vi "Drag Location.vi"(8 "error in (no error)":errorcluster, 9 "Coords":T4, 10 "BetterDropOp":refnum<class "BetterDropOp.lvclass">, 11 "Better Tree Handle In":refnum<class "BetterTreeHandle.lvclass">) -> (0 "error out":errorcluster, 2 "DragOver Output":T1={"Displayed Row"=0, "Position"=enum."On Row", "Row's TreeItem index"=0, "indent"=0, "Accepted?"=FALSE, "Insertion index"=0, "Top left visible TreeItem index"=0, "Bar type"=enum."tilda up"}, 3 "Better Tree Handle Out":refnum<class "BetterTreeHandle.lvclass">)   [LabVIEW 2020, in "BetterDragAndDrop.lvlib" / "BetterTreeHandle.lvclass"]
uses:
  BetterTreeHandle.lvclass
  <vilib>/Utility/miscctls.llb/LVPoint32TypeDef.ctl
  SubVIs/DragOver Output.ctl
  SubVIs/DragOverPosition.ctl
  BetterTreeBar/SubVIs/Horizontal Bar Enumeration.ctl
  C:/DSCE code/Open-source/betterdraganddrop_GIT/Source/Classes/BetterHandle/BetterHandle.lvclass
  BetterDropOp/BetterDropOp.lvclass
  BetterHandle/BetterHandle.lvclass/BetterHandle.ctl
  BetterTreeHandle.lvclass/BetterTreeHandle.ctl
  BetterTreeItem/BetterItem.lvclass
  BetterTreeBar/BetterHorizontalBar.lvclass
  BetterHandle/BetterHandle.lvclass
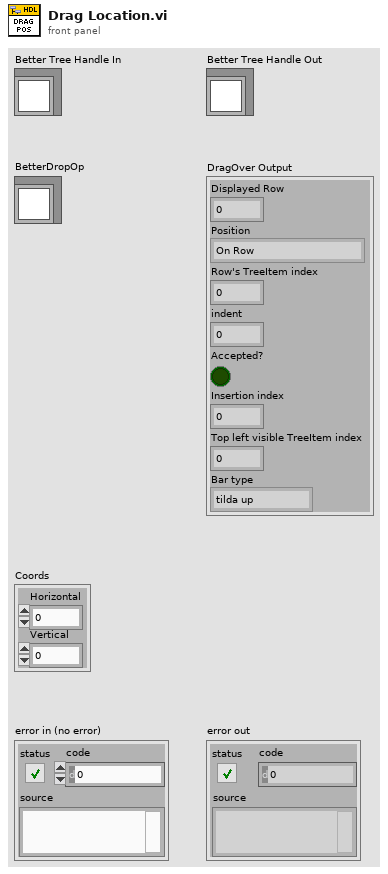
[diagram p1: front panel]
types:
  T1 = typedef "BetterDragAndDrop.lvlib/BetterHandle.lvclass/DragOver Output.ctl" = cluster{"Displayed Row":i32, "Position":T2, "Row's TreeItem index":i32, "indent":i32, "Accepted?":bool, "Insertion index":i32, "Top left visible TreeItem index":i32, "Bar type":T3}
  T2 = typedef "BetterDragAndDrop.lvlib/BetterHandle.lvclass/DragOverPosition.ctl" = enum16{"On Row", "Inbetween"}
  T3 = typedef "BetterDragAndDrop.lvlib/BetterHorizontalBar.lvclass/Horizontal Bar Enumeration.ctl" = enum16{"None", "only bar", "tilda up"}
  T4 = typedef "LVPoint32TypeDef.ctl" = cluster{"Horizontal":i32, "Vertical":i32}
  T5 = typedef "BetterDragAndDrop.lvlib/BetterHandle.lvclass/Pixel Constants.ctl" = cluster{"Row Header height":i32, "Row height":i32, "Column Header Offset":i32}
  T6 = typedef "BetterDragAndDrop.lvlib/BetterTreeHandle.lvclass/TreeItem.ctl" = cluster{"Left Cell String":string, "Child Text":string[], "Child Tag":string, "Item Indent":i32, "Child Only?":bool, "Glyph Index":i32, "Font Color":u32}
  T7 = typedef "LVPositionTypeDef.ctl" = cluster{"Left":i32, "Top":i32}
  T8 = typedef "LVNodeAndColumnTypeDef.ctl" = cluster{"Node":string, "Column":i32}
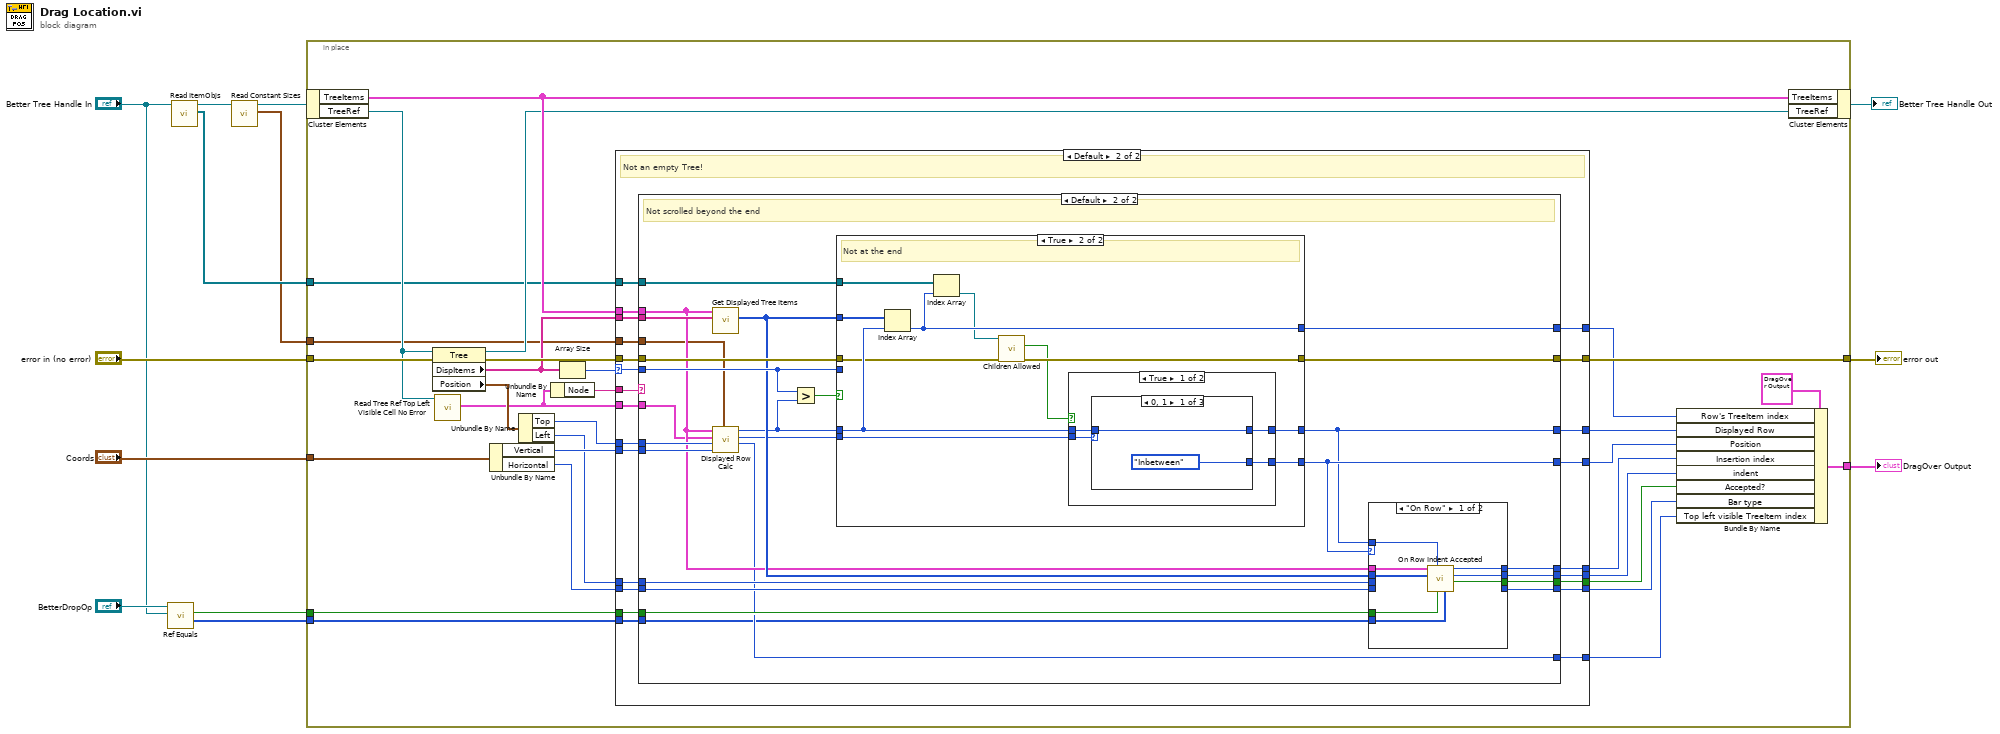
[diagram p0: block diagram]
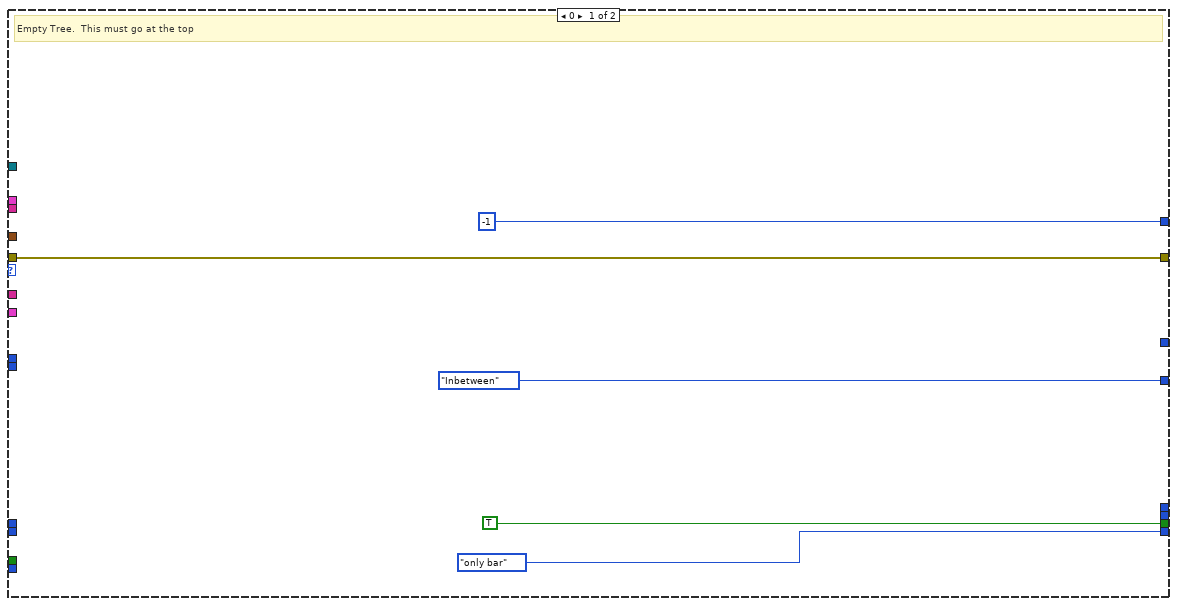
[diagram p2: hidden frame]
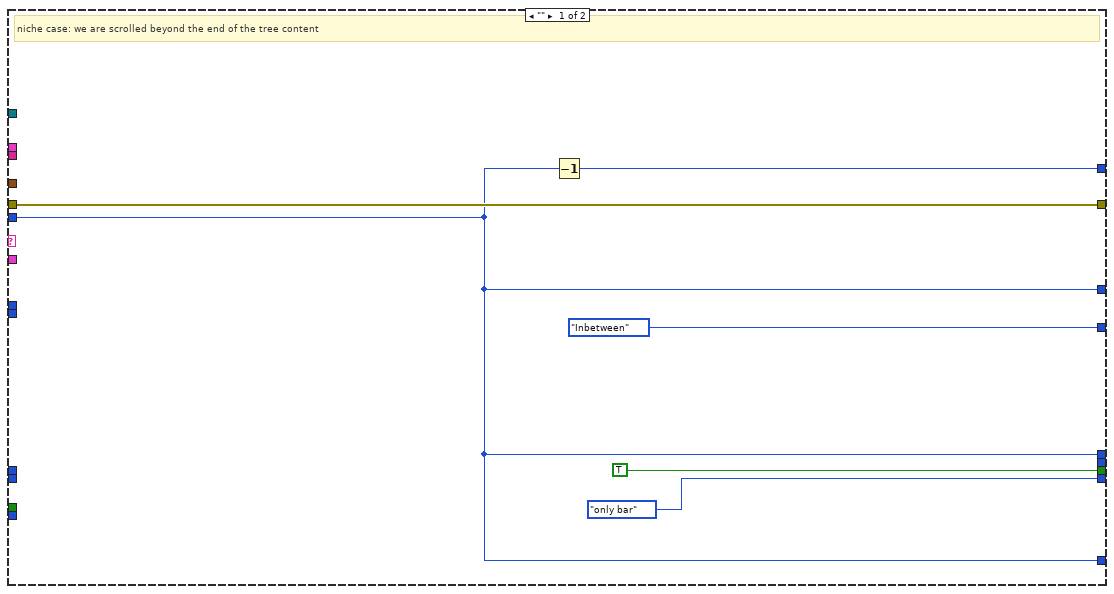
[diagram p3: hidden frame]
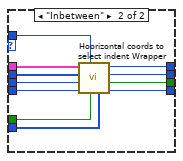
[diagram p4: hidden frame]
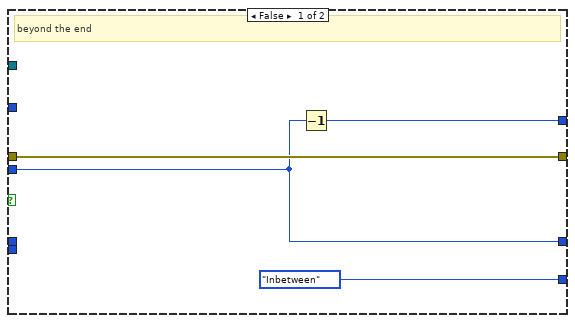
[diagram p5: hidden frame]
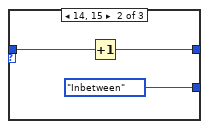
[diagram p6: hidden frame]
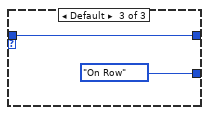
[diagram p7: hidden frame]
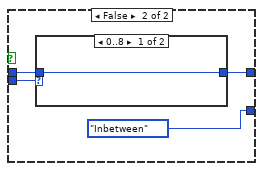
[diagram p8: hidden frame]
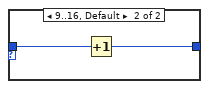
[diagram p9: hidden frame]
diagram:
  n1 = call "Ref Equals.vi"("BetterHandle in"="Better Tree Handle In", "BetterDropOp in"="BetterDropOp") -> ("DragStart Indices"=w8:i32[], "Ref is same?"=w7:bool)  [unwired: 6 in, 2 out]
  n2 = call "Read ItemObjs.vi"("BetterHandle in"="Better Tree Handle In") -> ("ItemObjs"=w4:refnum<class "BetterItem.lvclass">[], "BetterHandle out"=w3:refnum<class "BetterTreeHandle.lvclass">)  [unwired: 9 in]
  n3 = call "Read Constant Sizes.vi"("BetterHandle in"=w3) -> ("constant pixel sizes"=w1:T5, "BetterHandle out"=w2:refnum<class "BetterTreeHandle.lvclass">)  [unwired: 8 in, 1 out]
  n4 = in-place {
    in-place-border: "Coords" -> [w43]
    in-place-border: "error in (no error)" -> [w41]
    in-place-border: [w40] -> w10
    in-place-border: [w27] -> w11
    in-place-border: w8 -> [w17]
    in-place-border: w7 -> [w16]
    in-place-border: w4 -> [w15]
    in-place-border: w1 -> [w14]
    n5 = in-place-cluster #1(w2) -> ("TreeItems"=w36:T6[], "TreeRef"=w18:refnum<vi>)
    n6 = property class="Tree"(reference=w18, error in=w41) -> (reference out=w34:refnum<vi>, error out=w39:errorcluster, "DispItems"=w38:string[], "Position"=w25:T7)
    n7 = call "Read Tree Ref Top Left Visible Cell No Error.vi"("TreeRef"=w18) -> ("TopLeft"=w20:T8)  [unwired: 9 in, 1 out]
    n8 = Unbundle By Name(w43) -> ("Vertical"=w42:i32, "Horizontal"=w35:i32)
    n9 = Unbundle By Name(w25) -> ("Top"=w24:i32, "Left"=w23:i32)
    n10 = Unbundle By Name(w20) -> ("Node"=w19:string)
    n11 = Array Size(array=w38) -> (size(s)=w37:i32)
    n12 = case shown="Default" w37 {
      selector: w37 -> [_ w68]
      tunnel: w42 -> [_ w57]
      tunnel: [w48 w71] -> w40
      tunnel: w38 -> [_ w67]
      tunnel: w15 -> [_ w70]
      tunnel: w39 -> [w48 w69]
      tunnel: w24 -> [_ w56]
      tunnel: w36 -> [_ w55]
      tunnel: w35 -> [_ w66]
      tunnel: w23 -> [_ w65]
      tunnel: [_ w62] -> w32
      tunnel: [DragOverPosition."Inbetween" ("Position") w63] -> w31
      tunnel: [-1 w64] -> w30
      tunnel: w16 -> [_ w61]
      tunnel: [_ w60] -> w29
      tunnel: [_ w59] -> w28
      tunnel: [TRUE ("Allowed?") w58] -> w26
      tunnel: w20 -> [_ w54]
      tunnel: [_ w53] -> w22
      tunnel: [Horizontal_Bar_Enumeration."only bar" ("Bar type") w52] -> w21
      tunnel: w19 -> [_ w51]
      tunnel: w17 -> [_ w50]
      tunnel: w14 -> [_ w49]
      frame 0 {
        # "Empty Tree.  This must go at the top"
      }
      frame Default {
        # "Not an empty Tree!"
        n13 = case shown="Default" w51 {
          tunnel: [w73 w103] -> w71
          tunnel: w70 -> [_ w102]
          tunnel: w69 -> [w73 w101]
          tunnel: w68 -> [w72 w99]
          tunnel: w67 -> [_ w98]
          tunnel: w66 -> [_ w97]
          tunnel: w65 -> [_ w96]
          tunnel: [w74 w95] -> w64
          tunnel: [DragOverPosition."Inbetween" ("Position") w94] -> w63
          tunnel: [w72 w92] -> w62
          tunnel: w61 -> [_ w91]
          tunnel: [w72 w90] -> w60
          tunnel: [_ w89] -> w59
          tunnel: [TRUE ("Allowed?") w88] -> w58
          tunnel: w57 -> [_ w85]
          tunnel: w56 -> [_ w84]
          tunnel: w55 -> [_ w83]
          tunnel: w54 -> [_ w82]
          tunnel: [w72 w81] -> w53
          tunnel: [Horizontal_Bar_Enumeration."only bar" ("Bar type") w80] -> w52
          tunnel: w50 -> [_ w79]
          tunnel: w49 -> [_ w78]
          frame "" {
            # "niche case: we are scrolled beyond the end of the tree content"
            n14 = Decrement(x=w72) -> (x-1=w74:i32)
          }
          frame Default {
            # "Not scrolled beyond the end"
            n15 = call "Get Displayed Tree Items.vi"("Displayed Items"=w98, "TreeItems"=w83) -> ("TreeItem Indices (Displayed Items)"=w93:i32[])  [unwired: 8 in, 1 out]
            n16 = call "Displayed Row Calc.vi"("Constant Sizes"=w78, "Coords.Vertical"=w85, "Tree.Position:Top"=w84, "Top Left Visible Cell"=w82, "TreeItems"=w83) -> ("Top left visible TreeItem index"=w81:i32, "Pixels from top of row"=w86:i32, "Displayed Row"=w87:i32)  [unwired: 4 in]
            n17 = Greater?(x=w99, y=w87) -> (0:w100:bool)
            n18 = case shown="True" w100 {
              tunnel: w86 -> [_ w137]
              tunnel: [w126 w128] -> w103
              tunnel: w102 -> [_ w136]
              tunnel: w101 -> [w126 w129]
              tunnel: w87 -> [_ w134]
              tunnel: w99 -> [w124 _]
              tunnel: w93 -> [_ w135]
              tunnel: [w124 w133] -> w92
              tunnel: [DragOverPosition."Inbetween" ("Position") w132] -> w94
              tunnel: [w123 w131] -> w95
              frame False {
                # "beyond the end"
                n19 = Decrement(x=w124) -> (x-1=w123:i32)
              }
              frame True {
                # "Not at the end"
                n20 = Index Array(array=w135, index=w134) -> (element=w131:i32)
                n21 = Index Array(array=w136, index=w131) -> (element=w130:refnum<class "BetterItem.lvclass">)
                n22 = call-dynamic "Children Allowed.vi"("error in (no error)"=w129, "BetterTreeItem in"=w130) -> ("error out"=w128:errorcluster, "Child allowed?"=w127:bool)  [unwired: 7 in, 1 out]
                n23 = case shown="True" w127 {
                  tunnel: w137 -> [w141 w152]
                  tunnel: [w140 DragOverPosition."Inbetween" ("Position")] -> w132
                  tunnel: w134 -> [w139 w151]
                  tunnel: [w138 w150] -> w133
                  frame True {
                    n24 = case shown="0, 1" w141 {
                      tunnel: [DragOverPosition."Inbetween" ("Position") DragOverPosition."Inbetween" ("Position") DragOverPosition."On Row" ("Position")] -> w140
                      tunnel: w139 -> [w142 w145 w147]
                      tunnel: [w142 w144 w147] -> w138
                      frame 0, 1 {
                      }
                      frame 14, 15 {
                        n25 = Increment(x=w145) -> (x+1=w144:i32)
                      }
                      frame Default {
                      }
                    }
                  }
                  frame False {
                    n26 = case shown="0..8" w152 {
                      tunnel: w151 -> [w153 w155]
                      tunnel: [w153 w154] -> w150
                      frame 0..8 {
                      }
                      frame 9..16, Default {
                        n27 = Increment(x=w155) -> (x+1=w154:i32)
                      }
                    }
                  }
                }
              }
            }
            n28 = case shown="\"On Row\"" w94 {
              tunnel: w83 -> [w111 w122]
              tunnel: w97 -> [_ w119]
              tunnel: w96 -> [_ w120]
              tunnel: w93 -> [w108 w121]
              tunnel: w92 -> [w110 w117]
              tunnel: w91 -> [w109 w118]
              tunnel: [w107 w116] -> w90
              tunnel: [w106 w115] -> w89
              tunnel: [w105 w114] -> w88
              tunnel: [_ w113] -> w80
              tunnel: w79 -> [w104 w112]
              frame "On Row" {
                n29 = call "On Row Indent Accepted.vi"("DragStart.Drag Indices"=w104, "DragStart.DragOver Same?"=w109, "Displayed Row"=w110, "TreeItem Indices (Displayed Items)"=w108, "TreeItems"=w111) -> ("Allowed?"=w105:bool, "indent"=w106:i32, "Insertion index"=w107:i32)  [unwired: 4 in]
              }
              frame "Inbetween" {
                n30 = call "Hoorizontal coords to select indent Wrapper.vi"("DragStart.Drag Indices"=w112, "DragStart.DragOver Same?"=w118, "Displayed Row"=w117, "Coords.Horizontal"=w119, "Tree.Position:Left"=w120, "TreeItem Indices (Displayed Items)"=w121, "TreeItems"=w122) -> ("Bar type"=w113:T3, "Allowed?"=w114:bool, "indent"=w115:i32, "Insertion index"=w116:i32)  [unwired: 1 in]
              }
            }
          }
        }
      }
    }
    n31 = Bundle By Name(cluster=T1 {"Displayed Row"=9, "Position"=enum."Inbetween", "Row's TreeItem index"=8, "indent"=0, "Accepted?"=TRUE, "Insertion index"=0, "Top left visible TreeItem index"=0, "Bar type"=enum."tilda up"} ("Cluster"), "Row's TreeItem index"=w30, "Displayed Row"=w32, "Position"=w31, "Insertion index"=w29, "indent"=w28, "Accepted?"=w26, "Bar type"=w21, "Top left visible TreeItem index"=w22) -> (w27:T1)
    n32 = in-place-cluster #1("TreeItems"=w36, "TreeRef"=w34) -> (→"Better Tree Handle Out":refnum<class "BetterTreeHandle.lvclass">)
  }
  "error out" <- w10
  "DragOver Output" <- w11
